vi "Get First Available.vi"(10 "Column":string, 11 "Data In":T1) -> (2 "Index":i64, 3 "Value":string)   [LabVIEW 2020]
uses:
  Data.ctl
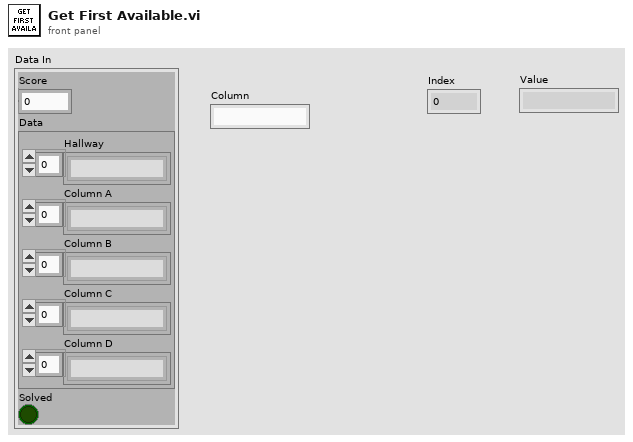
[diagram p1: front panel]
types:
  T1 = typedef "Data.ctl" = cluster{"Score":i64, "Data":cluster{"Hallway":string[], "Column A":string[], "Column B":string[], "Column C":string[], "Column D":string[]}, "Solved":bool}
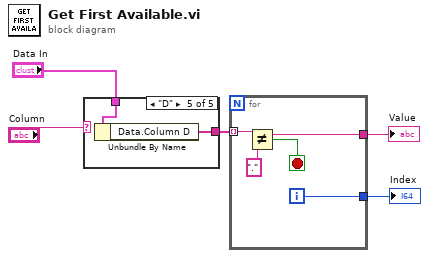
[diagram p0: block diagram]
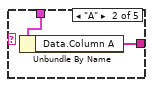
[diagram p3: hidden frame]
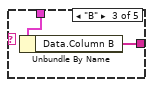
[diagram p4: hidden frame]
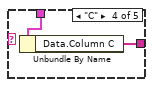
[diagram p5: hidden frame]
diagram:
  n1 = case shown="\"D\"" "Column" {
    tunnel: "Data In" -> [_ w7 w9 w11 w13]
    tunnel: [_ w6 w8 w10 w12] -> w3
    frame Default {
    }
    frame "A" {
      n2 = Unbundle By Name(w7) -> ("Data.Column A"=w6:string[])
    }
    frame "B" {
      n3 = Unbundle By Name(w9) -> ("Data.Column B"=w8:string[])
    }
    frame "C" {
      n4 = Unbundle By Name(w11) -> ("Data.Column C"=w10:string[])
    }
    frame "D" {
      n5 = Unbundle By Name(w13) -> ("Data.Column D"=w12:string[])
    }
  }
  n6 = for {
    tunnel: w3 -> [w15] mode=indexing
    tunnel: [w15] -> w1
    tunnel: [w14] -> w2
    i -> [w14]
    stop <- w16 stop-if-true
    n7 = Not Equal?(x=w15, y=".") -> (x != y?=w16:bool)
  }
  "Index" <- w2
  "Value" <- w1
